vi "E517_InitialisatOfWaveScan.vi"(0 "amplitude":dbl, 7 "Fast Axis":string="1", 8 "Slow Axis Steps":dbl, 11 "error in":errorcluster, 12 "FastAxisStepsize":dbl, 13 "kineticexposure":dbl) -> (4 "scan time for 1 line/sec":dbl=200.0 format="%.3g", 6 "scan time for 1 area/sec 2":dbl=200.0 format="%.3g", 15 "error out 2":errorcluster)   [LabVIEW 2011]
doc: "This VI initializes and configures the E-710 to perform a XY scan."
uses:
  Utilities/controls/ctlSeqFNs_PI_SysNr.ctl
  Variables/GlobalSetNumberOfDigits_PhysikalInstruments.vi
panel:
  out "Wavetable data":dbl[][](graph)
  out "Triggerpoints":dbl[][](graph)
  # "E-710 Wavescan Initialization"
  # "This VI initializes and configures the E-710 to perform a XY raster scan. Scan motion in X axis can be uni-\nor bidirectional. Triggerline 1 fires on waveform start."
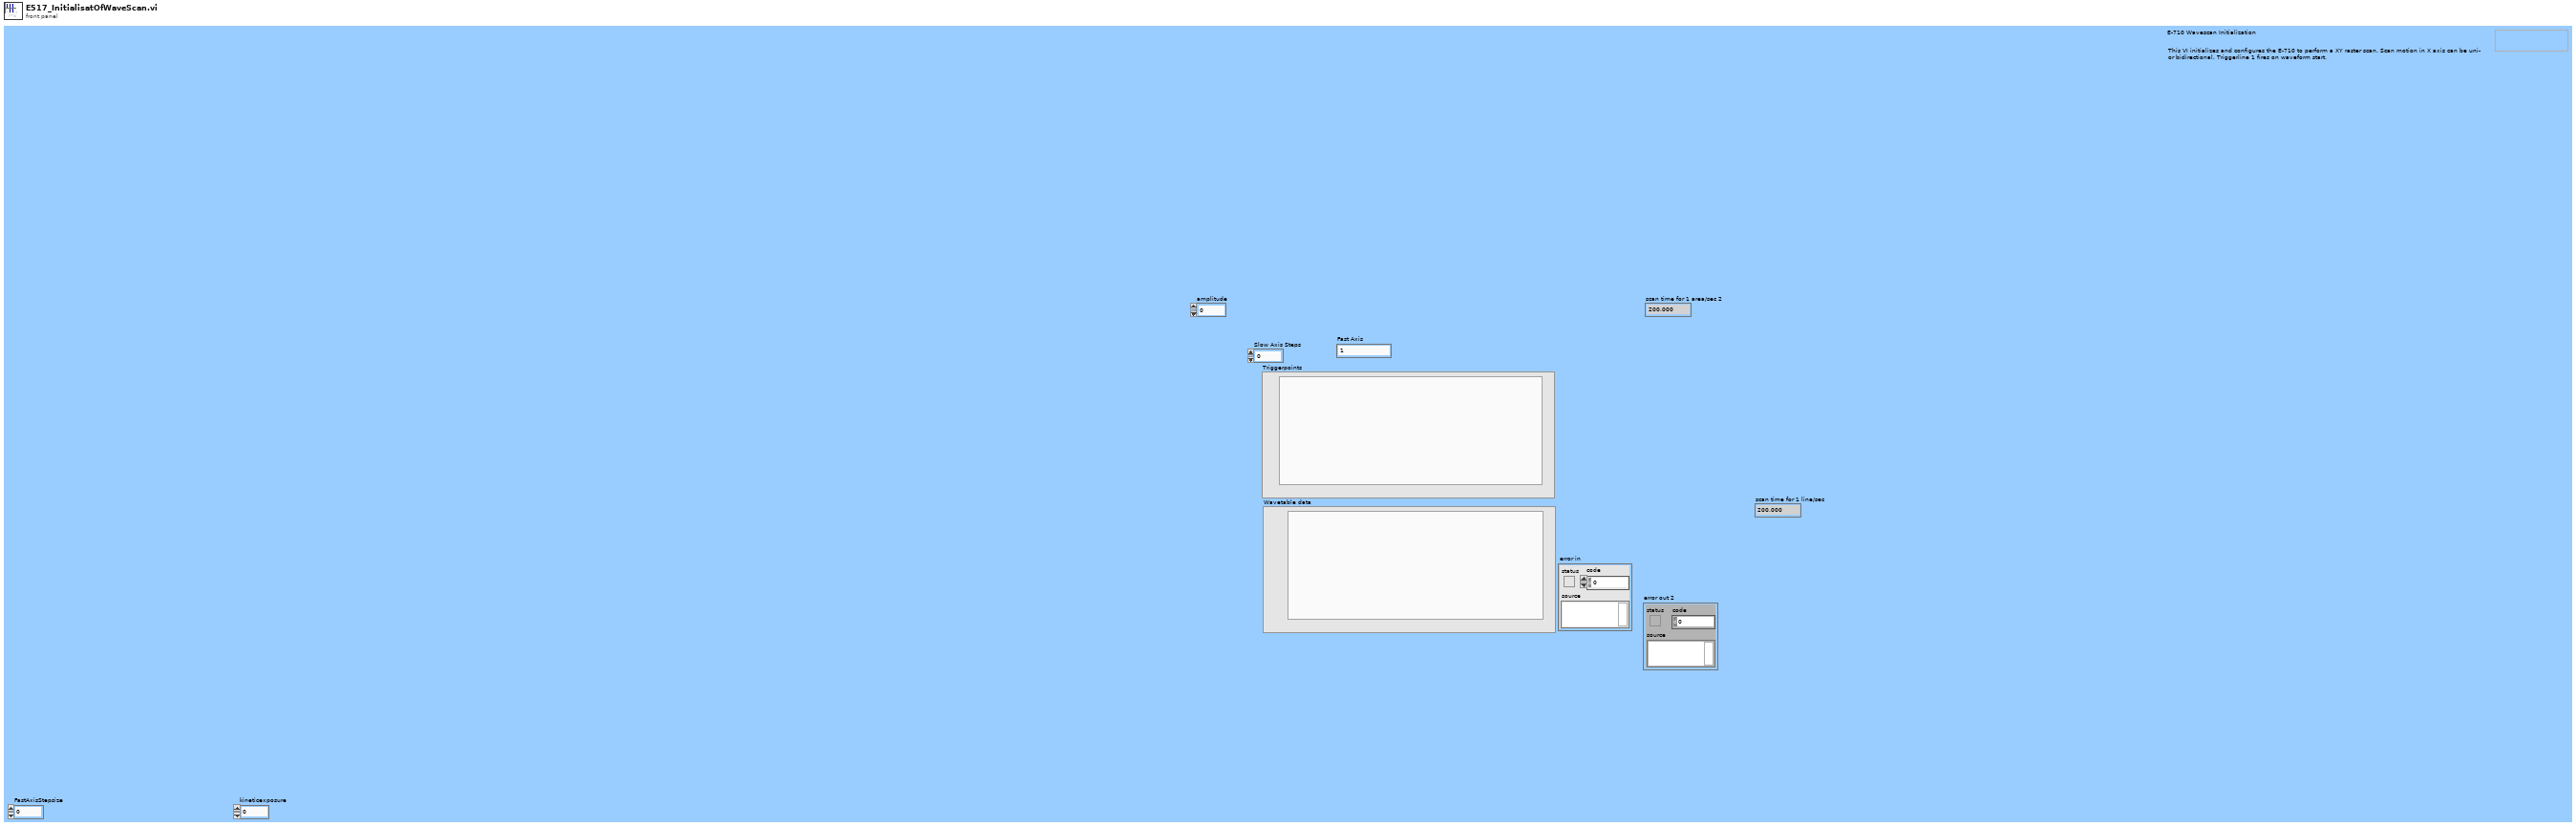
[diagram p1: front panel]
types:
  T1 = enum16{"Exit VI", "Set trigger mode", "Set recordtable rate", "Set wavetable rate", "Write sine", "Read wavetable", "Read recordtable", "Enable/disable wavegen", "Set number of wavegen cycles", "Clear wavetable", "Configure data recorder", "Assign wavetable to wavegen", "Read trigger points", "Set trigger points", "Clear trigger points", "Assign axes to triggerlines", "Write ramp waveform", "Set DDL enable", "Set DDL init", "Set Start at endpoint"}[]
  T2 = typedef "ctlSeqFNs_PI_SysNr.ctl" = enum16{"Zero", "E517", "E710"}
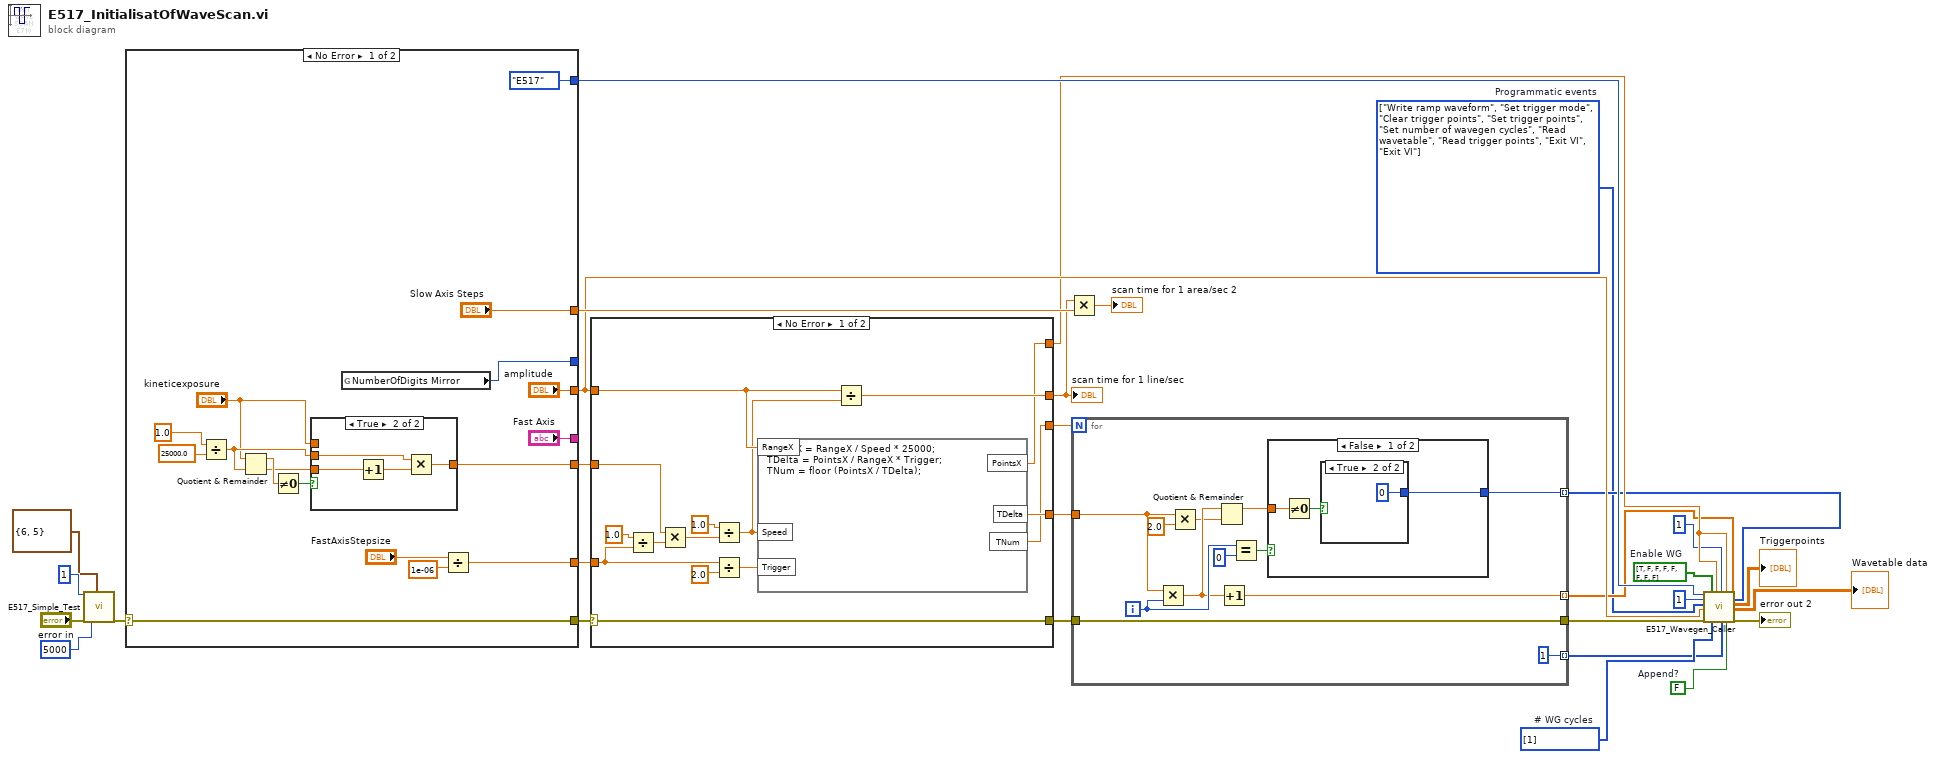
[diagram p0: block diagram]
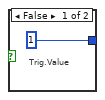
[diagram p2: hidden frame]
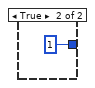
[diagram p3: hidden frame]
diagram:
  w7 = bool[] [TRUE, FALSE, FALSE, FALSE, FALSE, FALSE, FALSE, FALSE]  # Enable WG
  w5 = i32[] [1]  # # WG cycles
  w6 = FALSE  # Append?
  w1 = T1 [enum."Write ramp waveform", enum."Set trigger mode", enum."Clear trigger points", enum."Set trigger points", enum."Set number of wavegen cycles", enum."Read wavetable", enum."Read trigger points", enum."Exit VI", enum."Exit VI"] items=["Exit VI", "Set trigger mode", "Set recordtable rate", "Set wavetable rate", "Write sine", "Read wavetable", "Read recordtable", "Enable/disable wavegen", "Set number of wavegen cycles", "Clear wavetable", "Configure data recorder", "Assign wavetable to wavegen", "Read trigger points", "Set trigger points", "Clear trigger points", "Assign axes to triggerlines", "Write ramp waveform", "Set DDL enable", "Set DDL init", "Set Start at endpoint"]  # Programmatic events
  n1 = call "E517_Simple_Test.vi"("System no."=1, "error in"="error in", "Timeout"=u32 5000, "RS232 settings"=cluster{"Portnumber":i32, "Baudrate":u16} {"Portnumber"=6, "Baudrate"=5}) -> ("error out"=w16:errorcluster)  [unwired: 11 in, 4 out]
  n2 = case shown="No Error" w16 {
    selector: w16 -> [w43 w53]
    tunnel: ["Fast Axis" _] -> _
    tunnel: [ctlSeqFNs_PI_SysNr."E517" ("STATE") _] -> w26
    tunnel: [w45 _] -> _
    tunnel: ["Slow Axis Steps" _] -> w30
    tunnel: [w43 w53] -> w28
    tunnel: ["amplitude" _] -> w21
    tunnel: [w40 _] -> w29
    tunnel: [w32 _] -> w25
    frame No Error {
      n3 = Divide(x=1.0, y=25000.0) -> (x/y=w33:dbl)
      n4 = Quotient & Remainder(x="kineticexposure", y=w33) -> (x-y*floor(x/y)=w36:dbl, floor(x/y)=w34:dbl)
      n5 = Not Equal To 0?(x=w36) -> (x != 0?=w35:bool)
      n6 = case shown="True" w35 {
        tunnel: w34 -> [_ w52]
        tunnel: w33 -> [_ w50]
        tunnel: [w48 w49] -> w32
        tunnel: "kineticexposure" -> [w48 _]
        frame False {
        }
        frame True {
          n7 = Increment(x=w52) -> (x+1=w51:dbl)
          n8 = Multiply(x=w50, y=w51) -> (x*y=w49:dbl)
        }
      }
      n9 = global read "GlobalSetNumberOfDigits_PhysikalInstruments.vi" "NumberOfDigits Mirror"() -> (w45:i32)
      n10 = Divide(x="FastAxisStepsize", y=1e-06) -> (x/y=w40:dbl)
    }
    frame Error {
    }
  }
  n11 = case shown="No Error" w28 {
    selector: w28 -> [w67 _]
    tunnel: [w68 _] -> w23
    tunnel: w21 -> [w61 _]
    tunnel: w29 -> [w58 _]
    tunnel: [w54 _] -> w18
    tunnel: [w67 _] -> w22
    tunnel: [w66 _] -> w27
    tunnel: w25 -> [w59 _]
    tunnel: [w55 _] -> w24
    frame No Error {
      n12 = Divide(x=1.0, y=w58) -> (x/y=w64:dbl)
      n13 = Multiply(x=w59, y=w64) -> (x*y=w63:dbl)
      n14 = Divide(x=1.0, y=w63) -> (x/y=w60:dbl)
      n15 = Divide(x=w58, y=2.0) -> (x/y=w56:dbl)
      n16 = formula code="PointsX = RangeX / Speed * 25000;\nTDelta = PointsX / RangeX * Trigger;\nTNum = floor (PointsX / TDelta);"("RangeX"=w61, "Speed"=w60, "Trigger"=w56) -> ("PointsX"=w54:dbl, "TDelta"=w68:dbl, "TNum"=w55:dbl)
      n17 = Divide(x=w61, y=w60) -> (x/y=w66:dbl)
    }
    frame Error {
    }
  }
  "scan time for 1 line/sec" <- w27
  n18 = Multiply(x=w27, y=w30) -> (x*y=→"scan time for 1 area/sec 2":dbl)
  n19 = for {
    N: w24 -> [_]
    tunnel: w23 -> [w74]
    tunnel: [w71] -> w2 mode=indexing
    tunnel: [w80] -> w4 mode=indexing
    tunnel: w22 -> [w76]
    tunnel: [w76] -> w10
    tunnel: [1] -> w3 mode=indexing
    i -> [w72]
    n20 = Multiply(x=w74, y=w72) -> (x*y=w70:dbl)
    n21 = Multiply(x=w74, y=2.0) -> (x*y=w69:dbl)
    n22 = Quotient & Remainder(x=w70, y=w69) -> (x-y*floor(x/y)=w79:dbl)  [unwired: 1 out]
    n23 = Increment(x=w70) -> (x+1=w71:dbl)
    n24 = Equal?(x=w72, y=0) -> (x = y?=w77:bool)
    n25 = case shown="False" w77 {
      tunnel: [w83 1] -> w80
      tunnel: w79 -> [w82 _]
      frame False {
        n26 = Not Equal To 0?(x=w82) -> (x != 0?=w81:bool)
        n27 = case shown="True" w81 {
          tunnel: [1 0] -> w83
          frame False {
            # "Trig.Value"
          }
          frame True {
          }
        }
      }
      frame True {
      }
    }
  }
  n28 = call "E517_Wavegen_Caller.vi"("System no."=w26, "# Wavegenerators"=1, "Programmatic events"=w1, "FastAxisLength"=w21, "error in"=w10, "Enabled"=w7, "# WG cycles"=w5, "N"=w18, "Xo"=1, "TriggerVal"=w3, "Segm.Length"=w18, "Append?"=w6, "Wavepoint"=w2, "Switch"=w4) -> ("Triggerpoints"=→"Triggerpoints":dbl[][], "Wavetable data"=→"Wavetable data":dbl[][], "Error out"=→"error out 2":errorcluster)  [unwired: 2 in, 1 out]
